vi "GUILib.simple numeric change increment.vi"(0 "ctlRef":refnum<vi>, 2 "increment":dbl, 5 "error in (no error)":errorcluster) -> (14 "ctlRef dup":refnum<vi>, 19 "error out":errorcluster)   [LabVIEW 2012, in "GUILib.lvlib"]
doc: "changes the increment value for a specific type of control"
uses:
  GUILib.lvlib
  GUILib.simpleNumeric.ctl
  GUILib.basicNumeric.ctl
panel:
  in  "simpleNumericType":T1 {"nom" step=22.0}
  in  "numericType":dbl
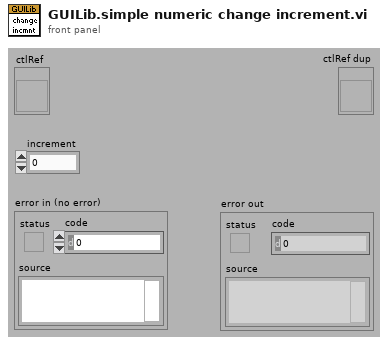
[diagram p1: front panel]
types:
  T1 = typedef "GUILib.lvlib/GUILib.simpleNumeric.ctl" = cluster{"nom":T2, "act":dbl, "inc":dbl}
  T2 = typedef "GUILib.lvlib/GUILib.basicNumeric.ctl" = dbl
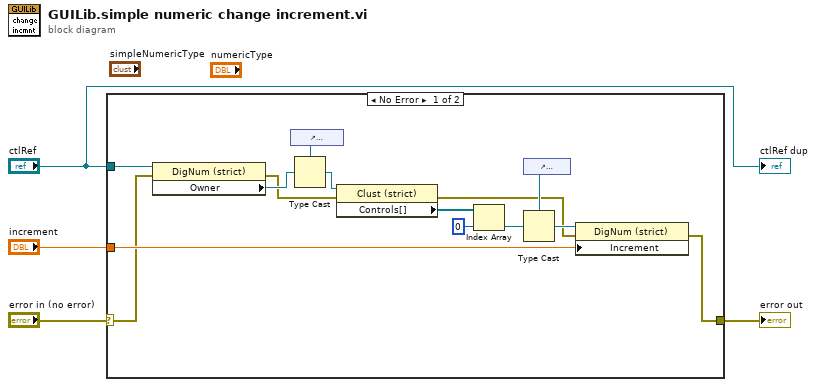
[diagram p0: block diagram]
diagram:
  n1 = case shown="No Error" "error in (no error)" {
    selector: "error in (no error)" -> [w8 w19]
    tunnel: "increment" -> [w18 _]
    tunnel: "ctlRef" -> [w11 _]
    tunnel: [w5 w19] -> w1
    frame No Error {
      n2 = property on="Property Node" class="DigNum (strict)"(reference=w11, error in=w8) -> (error out=w7:errorcluster, "Owner"=w12:refnum<vi>)  [unwired: 1 out]
      n3 = control-ref of="simpleNumericType"() -> (w9:refnum<vi>)
      n4 = Type Cast(type=w9, x=w12) -> (*(type *) &x=w13:refnum<vi>)
      n5 = property on="Property Node" class="Clust (strict)"(reference=w13, error in=w7) -> (error out=w6:errorcluster, "Controls[]"=w14:refnum<vi>[])  [unwired: 1 out]
      n6 = Index Array(array=w14, index=0) -> (element=w16:refnum<vi>)
      n7 = control-ref of="numericType"() -> (w10:refnum<vi>)
      n8 = Type Cast(type=w10, x=w16) -> (*(type *) &x=w17:refnum<vi>)
      n9 = property on="Property Node" class="DigNum (strict)"(reference=w17, error in=w6, "Increment"=w18) -> (error out=w5:errorcluster)  [unwired: 1 out]
    }
    frame Error {
    }
  }
  "error out" <- w1
  "ctlRef dup" <- "ctlRef"
